vi "handle error.vi"(8 "error in":errorcluster, 11 "communicator in":refnum<class "communicator.lvclass">) -> (0 "unrecoverable?":bool, 3 "communicator out":refnum<class "communicator.lvclass">)   [LabVIEW 2015, in "communicator.lvclass"]
uses:
  communicator.lvclass
  communicator queue/enqueue variety.ctl
  message/communicator message.lvclass/communicator message.ctl
  communicator.lvclass/communicator.ctl
  communicator queue/identifying queue.lvclass/identifying queue.ctl
  message/create message.vi
  communicator queue/send.vi
  message/set sender.vi
  message/communicator message.lvclass
  communicator queue/identifying queue.lvclass
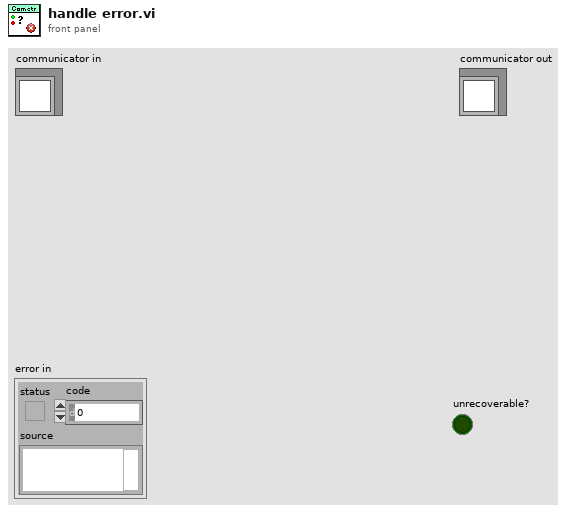
[diagram p1: front panel]
types:
  T1 = typedef "identifying queue.lvclass/enqueue variety.ctl" = enum16{"normal", "lossy", "priority"}
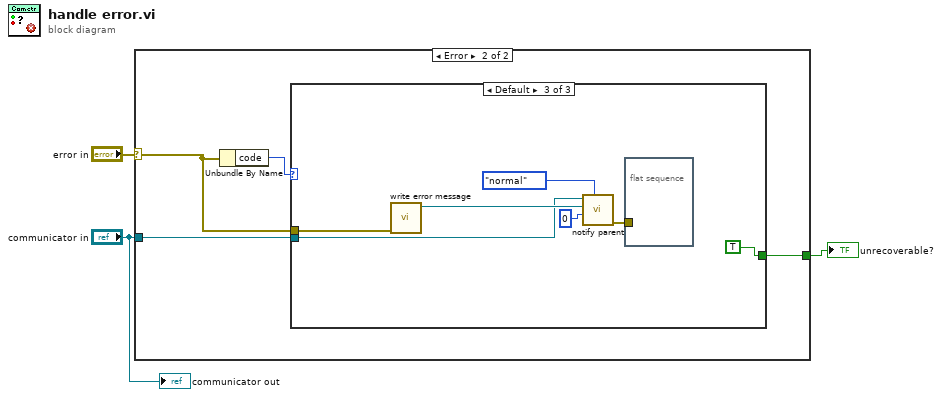
[diagram p0: block diagram]
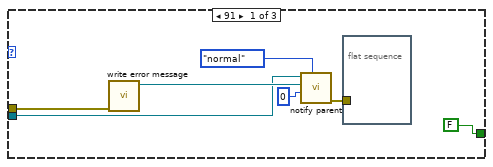
[diagram p3: hidden frame]
diagram:
  n1 = case shown="Error" "error in" {
    selector: "error in" -> [_ w6]
    tunnel: "communicator in" -> [_ w7]
    tunnel: [_ w4] -> w1
    frame No Error {
    }
    frame Error {
      n2 = Unbundle By Name(w6) -> ("code"=w5:i32)
      n3 = case shown="Default" w5 {
        tunnel: w7 -> [w13 _ w20]
        tunnel: w6 -> [w9 _ w16]
        tunnel: [FALSE _ TRUE] -> w4
        frame 91 {
          n4 = call "write error message.vi"("error in"=w9) -> ("element"=w14:refnum<class "communicator message.lvclass">)  [unwired: 10 in]
          n5 = call "notify parent.vi"("enqueue setting"=enqueue_variety."normal", "timeout in ms (-1)"=0, "element"=w14, "communicator in"=w13) -> ("error out"=w10:errorcluster)  [unwired: 7 in]
          n6 = flat-sequence {
            tunnel: w10 -> [_]
            frame #0 {
            }
          }
        }
        frame 590000..590002 {
        }
        frame Default {
          n7 = call "write error message.vi"("error in"=w16) -> ("element"=w21:refnum<class "communicator message.lvclass">)  [unwired: 10 in]
          n8 = call "notify parent.vi"("enqueue setting"=enqueue_variety."normal", "timeout in ms (-1)"=0, "element"=w21, "communicator in"=w20) -> ("error out"=w17:errorcluster)  [unwired: 7 in]
          n9 = flat-sequence {
            tunnel: w17 -> [_]
            frame #0 {
            }
          }
        }
      }
    }
  }
  "unrecoverable?" <- w1
  "communicator out" <- "communicator in"
